vi "channel pairing test.vi"() -> (0 "error out":errorcluster, 3 "Data allocations match?":bool)   [LabVIEW 2015, in "E2E Tag Exchange tests.lvlib"]
uses:
  E2E Tag Exchange tests.lvlib
  <vilib>/NI/Module Execution Interface/Engine Configuration/engine configuration.lvclass
  <vilib>/NI/Configuration Framework/serializable configuration/NISE_CEF_serializable configuration.lvclass/NISE_CEF_serializable configuration.ctl
  <vilib>/Utility/LVClass/Get LV Class Name.vi
  <vilib>/NI/Configuration Framework/error generator/NISE_error generator.vi
  module/configuration/E2E Tag Exchange configuration.lvclass
  <vilib>/NI/Tag Bus Module Framework/channel/TBM channel.lvclass
  <vilib>/NI/Configuration Framework/serializable configuration/NISE_CEF_serializable configuration.lvclass
  editor node/E2E Tag Exchange editor node.lvclass
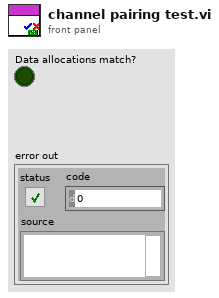
[diagram p1: front panel]
types:
  T1 = typedef "TBM channel.lvclass/data tables.ctl" = cluster{"input data":T2, "processing parameter":T2, "processing result":T2, "output data":T2}
  T2 = typedef "tag bus.lvlib/dictionary table pair.ctl" = cluster{"data dictionary":refnum<class "data dictionary.lvclass">, "data table":T3}
  T3 = typedef "tag bus.lvlib/data table.lvlib/data table.ctl" = cluster{"Double":dbl[], "Single":sgl[], "I64":i64[], "I32":i32[], "I16":i16[], "I8":i8[], "U64":u64[], "U32":u32[], "U16":u16[], "U8":u8[], "Boolean":bool[], "String":string[], "Array of Double":cluster{"DBL Array":dbl[]}[], "Array of Single":cluster{"SGL Array":sgl[]}[], "Array of I64":cluster{"I64 Array":i64[]}[], "Array of I32":cluster{"I32 Array":i32[]}[], "Array of I16":cluster{"I16 Array":i16[]}[], "Array of I8":cluster{"I8 Array":i8[]}[], "Array of U64":cluster{"U64 Array":u64[]}[], "Array of U32":cluster{"U32 Array":u32[]}[], "Array of U16":cluster{"U16 Array":u16[]}[], "Array of U8":cluster{"U8 Array":u8[]}[], "Array of Boolean":cluster{"Boolean Array":bool[]}[], "Array of String":cluster{"String Array":string[]}[]}
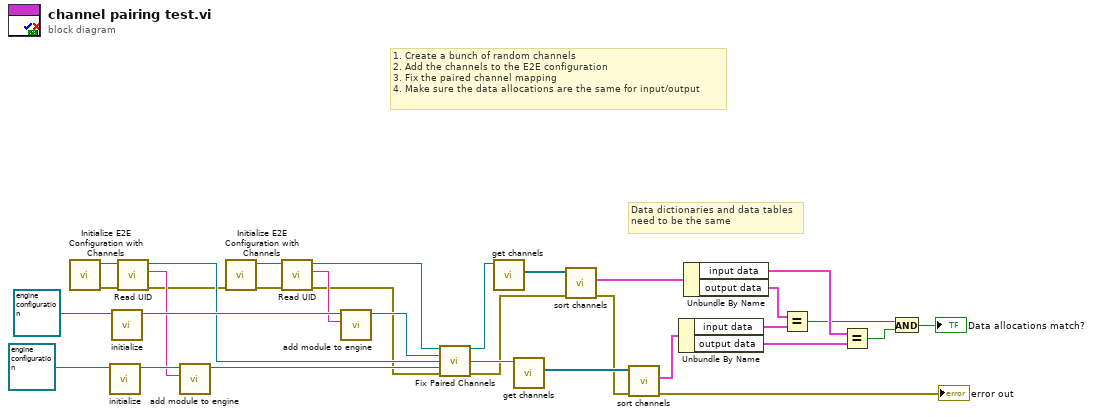
[diagram p0: block diagram]
diagram:
  # "1. Create a bunch of random channels\n2. Add the channels to the E2E configuration\n3. Fix the paired channel mapping\n4. Make sure the data allocations are the same for input/output"
  # "Data dictionaries and data tables\nneed to be the same"
  n1 = call "Initialize E2E Configuration with Channels.vi"() -> ("error out"=w9:errorcluster, "Initialized E2E configuration"=w10:refnum<class "E2E Tag Exchange configuration.lvclass">)  [unwired: 9 in, 1 out]
  n2 = call <vilib>:"initialize.vi"("configuration in"=refnum<class "engine configuration.lvclass"> refnum ("engine configuration")) -> ("configuration out"=w25:refnum<class "engine configuration.lvclass">)  [unwired: 8 in, 2 out]
  n3 = call <vilib>:"initialize.vi"("configuration in"=refnum<class "engine configuration.lvclass"> refnum ("engine configuration")) -> ("configuration out"=w26:refnum<class "engine configuration.lvclass">)  [unwired: 8 in, 2 out]
  n4 = call <vilib>:"Read UID.vi"("error in"=w9, "configuration in"=w10) -> ("error out"=w3:errorcluster, "instance id"=w5:string, "configuration out"=w4:refnum<class "E2E Tag Exchange configuration.lvclass">)  [unwired: 7 in]
  n5 = call-dynamic "add module to engine.vi"("module ID"=w5, "engine configuration in"=w25) -> ("engine configuration out"=w15:refnum<class "engine configuration.lvclass">)  [unwired: 8 in, 1 out]
  n6 = call "Initialize E2E Configuration with Channels.vi"("error in"=w3) -> ("error out"=w7:errorcluster, "Initialized E2E configuration"=w8:refnum<class "E2E Tag Exchange configuration.lvclass">)  [unwired: 8 in, 1 out]
  n7 = call <vilib>:"Read UID.vi"("error in"=w7, "configuration in"=w8) -> ("error out"=w1:errorcluster, "instance id"=w6:string, "configuration out"=w2:refnum<class "E2E Tag Exchange configuration.lvclass">)  [unwired: 7 in]
  n8 = call-dynamic "add module to engine.vi"("module ID"=w6, "engine configuration in"=w26) -> ("engine configuration out"=w14:refnum<class "engine configuration.lvclass">)  [unwired: 8 in, 1 out]
  n9 = call "Fix Paired Channels.vi"("Paired E2E configuration in"=w2, "Paired engine configuration in"=w14, "E2E configuration in"=w4, "engine configuration in"=w15, "error in (no error)"=w1) -> ("Paired E2E configuration out"=w17:refnum<class "E2E Tag Exchange configuration.lvclass">, "E2E configuration out"=w16:refnum<class "E2E Tag Exchange configuration.lvclass">, "error out"=w13:errorcluster)  [unwired: 6 in, 2 out]
  n10 = call-dynamic "get channels.vi"("E2E configuration in"=w17) -> ("channels"=w32:refnum<class "TBM channel.lvclass">[])  [unwired: 9 in, 1 out]
  n11 = call-dynamic "get channels.vi"("E2E configuration in"=w16) -> ("channels"=w31:refnum<class "TBM channel.lvclass">[])  [unwired: 9 in, 1 out]
  n12 = call <vilib>:"sort channels.vi"("error in"=w13, "channels in"=w32) -> ("error out"=w12:errorcluster, "data allocations"=w30:T1)  [unwired: 7 in, 1 out]
  n13 = call <vilib>:"sort channels.vi"("error in"=w12, "channels in"=w31) -> ("error out"=→"error out":errorcluster, "data allocations"=w29:T1)  [unwired: 7 in, 1 out]
  n14 = Unbundle By Name(w29) -> ("input data"=w21:T2, "output data"=w23:T2)
  n15 = Unbundle By Name(w30) -> ("input data"=w24:T2, "output data"=w22:T2)
  n16 = Equal?(x=w22, y=w21) -> (x = y?=w20:bool)
  n17 = Equal?(x=w24, y=w23) -> (x = y?=w19:bool)
  n18 = And(x=w20, y=w19) -> (x .and. y?=→"Data allocations match?":bool)
